vi "pc_write_cond_2.vi"(0 "X":dbl[](array[numeric]), 2 "Count In":i32, 3 "Max Count":i32=2, 5 "Y":dbl[](array[numeric]), 7 "Touch 1":bool[](array[boolean]), 9 "Touch 2":bool[](array[boolean]), 11 "Nose Poke":bool[](array[boolean]), 12 "Dispense":bool[](array[boolean]), 13 "Opto On":bool[](array[boolean])) -> (4 "Write Current":bool, 6 "Write Previous":bool, 8 "Current Data":string, 10 "Previous Data":string, 15 "Count Out":i32)   [LabVIEW 2013]
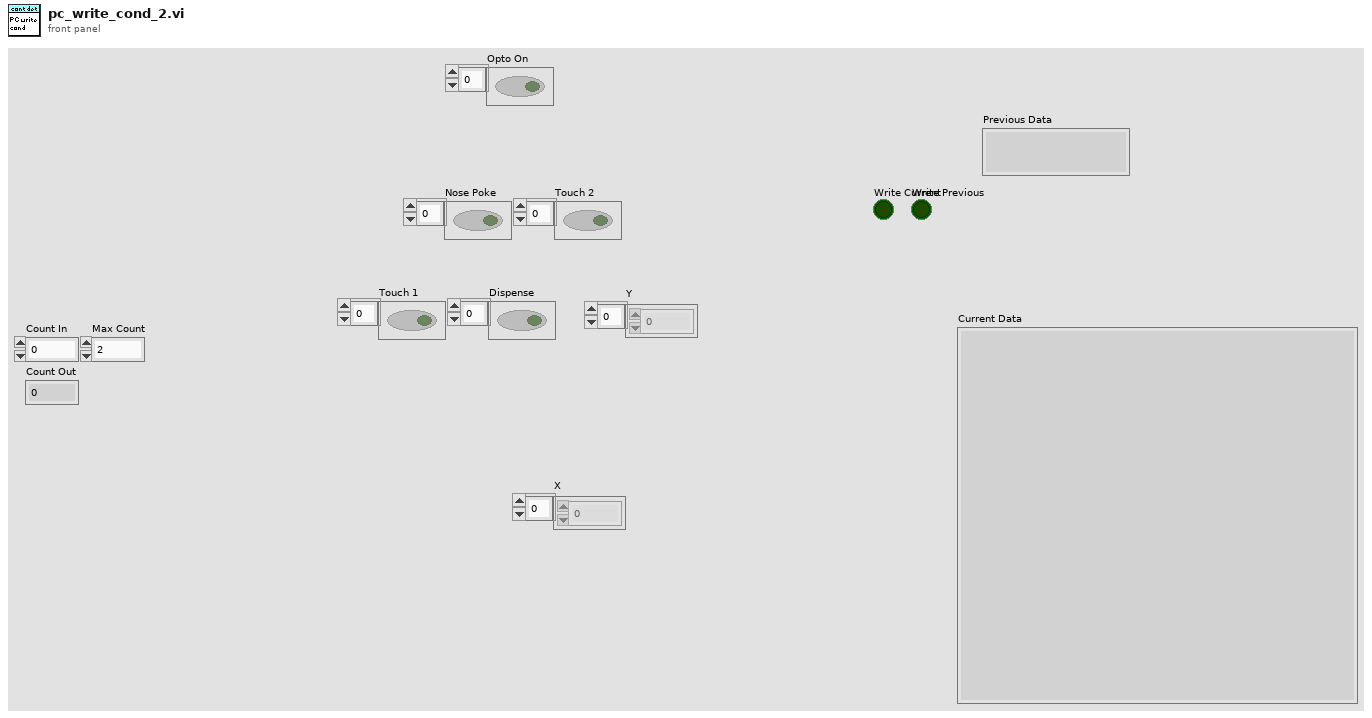
[diagram p1: front panel]
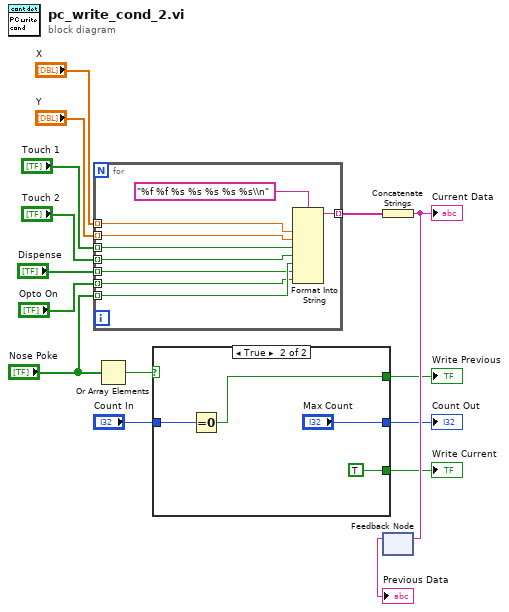
[diagram p0: block diagram]
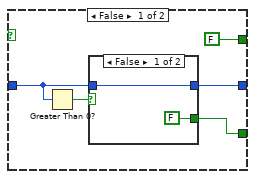
[diagram p2: hidden frame]
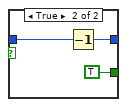
[diagram p3: hidden frame]
diagram:
  n1 = for {
    tunnel: "X" -> [w24] mode=indexing
    tunnel: "Y" -> [w23] mode=indexing
    tunnel: "Touch 1" -> [w22] mode=indexing
    tunnel: "Touch 2" -> [w21] mode=indexing
    tunnel: "Nose Poke" -> [w20] mode=indexing
    tunnel: "Dispense" -> [w19] mode=indexing
    tunnel: [w17] -> w8 mode=indexing
    tunnel: "Opto On" -> [w16] mode=indexing
    n2 = Format Into String(format string="%f %f %s %s %s %s %s\\n", w24, w23, w22, w21, w20, w19, w16) -> (resulting string=w17:string)  [unwired: 2 in, 1 out]
  }
  n3 = Or Array Elements(Boolean array="Nose Poke") -> (logical OR=w2:bool)
  n4 = case shown="True" w2 {
    tunnel: "Count In" -> [w28 w38]
    tunnel: [w27 "Max Count"] -> w5
    tunnel: [FALSE w36] -> w4
    tunnel: [w26 TRUE] -> w3
    frame False {
      n5 = Greater Than 0?(x=w28) -> (x > 0?=w29:bool)
      n6 = case shown="False" w29 {
        tunnel: w28 -> [w31 w34]
        tunnel: [w31 w33] -> w27
        tunnel: [FALSE TRUE] -> w26
        frame False {
        }
        frame True {
          n7 = Decrement(x=w34) -> (x-1=w33:i32)
        }
      }
    }
    frame True {
      n8 = Equal To 0?(x=w38) -> (x = 0?=w36:bool)
    }
  }
  "Write Current" <- w3
  "Count Out" <- w5
  "Write Previous" <- w4
  n9 = Concatenate Strings(w8) -> (w7:string)
  "Current Data" <- w7
  n10 = feedback #1() -> (→"Previous Data":string)  [unwired: 1 in]
  n11 = feedback-in #1(w7) -> ()
